vi "Sift Bob's Key.vi"(8 "error in":errorcluster, 10 "PM Level in":u8[](array[numeric]), 11 "SPD Number in":u8[](array[numeric])) -> (0 "error out":errorcluster, 2 "Sifted Bob's data":u32[](array[numeric]), 3 "Raw Bob's data":u8[](array[numeric]))   [LabVIEW 2018]
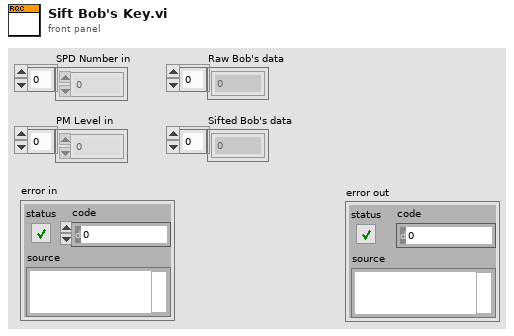
[diagram p1: front panel]
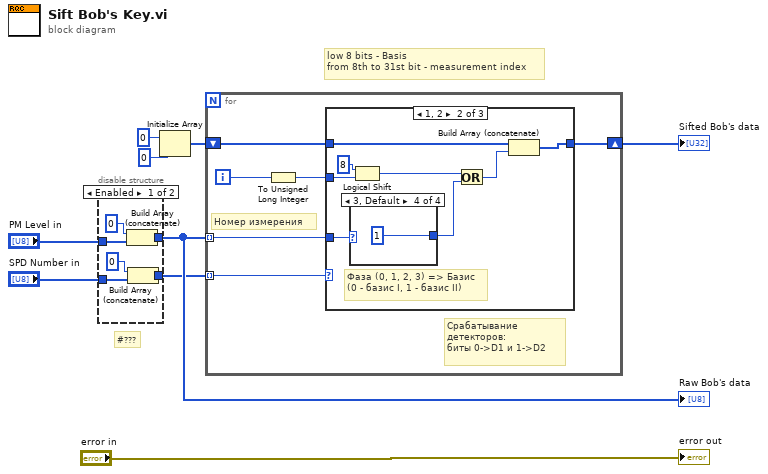
[diagram p0: block diagram]
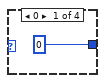
[diagram p4: hidden frame]
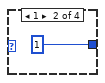
[diagram p5: hidden frame]
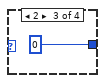
[diagram p6: hidden frame]
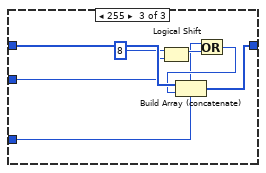
[diagram p7: hidden frame]
diagram:
  # "#???"
  # "low 8 bits - Basis\nfrom 8th to 31st bit - measurement index"
  n1 = disable-structure shown="Enabled" {
    disable-tunnel: "PM Level in" -> [w15 w17]
    disable-tunnel: [w14 w17] -> w4
    disable-tunnel: "SPD Number in" -> [w11 w16]
    disable-tunnel: [w10 w16] -> w2
    frame Enabled {
      n2 = Build Array (concatenate)(u8 0, w15) -> (w14:u8[])
      n3 = Build Array (concatenate)(u8 0, w11) -> (w10:u8[])
    }
    frame Disabled {
    }
  }
  "Raw Bob's data" <- w4
  n4 = Initialize Array(u32 0, 0 ("dimension size")) -> (w7:u32[])
  n5 = for {
    shift-right: [w23] -> w1
    shift-left: w7 -> [w22]
    tunnel: w4 -> [w20] mode=indexing
    tunnel: w2 -> [w21] mode=indexing
    i -> [w18]
    # "Срабатывание детекторов:\nбиты 0->D1 и 1->D2"
    # "Номер измерения"
    n6 = To Unsigned Long Integer(number=w18) -> (unsigned 32bit integer=w19:u32)
    n7 = case shown="1, 2" w21 {
      tunnel: [w24 w29 w42] -> w23
      tunnel: w22 -> [w24 w27 w43]
      tunnel: w19 -> [_ w28 w41]
      tunnel: w20 -> [_ w25 w37]
      frame 0, Default {
      }
      frame 1, 2 {
        # "Фаза (0, 1, 2, 3) => Базис (0 - базис I, 1 - базис II)"
        n8 = case shown="3, Default" w25 {
          tunnel: [u32 0 u32 1 u32 0 u32 1] -> w26
          frame 0 {
          }
          frame 1 {
          }
          frame 2 {
          }
          frame 3, Default {
          }
        }
        n9 = Logical Shift(y=8, x=w28) -> (x << y=w31:u32)
        n10 = Or(x=w31, y=w26) -> (x .or. y?=w30:u32)
        n11 = Build Array (concatenate)(w27, w30) -> (w29:u32[])
      }
      frame 255 {
        n12 = Logical Shift(y=8, x=w41) -> (x << y=w39:u32)
        n13 = Or(x=w37, y=w39) -> (x .or. y?=w38:u32)
        n14 = Build Array (concatenate)(w43, w38) -> (w42:u32[])
      }
    }
  }
  "Sifted Bob's data" <- w1
  "error out" <- "error in"
